vi "EI1050 Config.vi"(6 "Power Channel":i32=2, 7 "Enable Channels":i32[](array[numeric]), 8 "error in":errorcluster, 9 "Clock Channel":i32=1, 10 "Data Channel":i32, 11 "Handle In":i32) -> (0 "error out":errorcluster, 3 "Handle Out":i32)   [LabVIEW 2021]
panel:
  # "This array can be left empty if\nthere is only 1 EI-1050 and enable/disable\nis not needed."
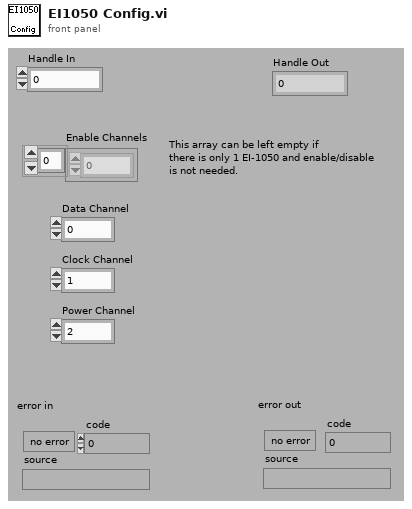
[diagram p1: front panel]
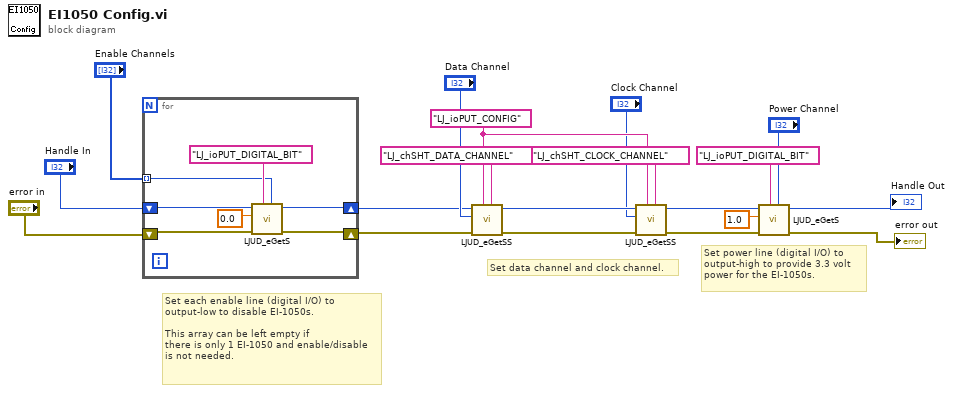
[diagram p0: block diagram]
diagram:
  w17 = "LJ_ioPUT_CONFIG"
  # "Set power line (digital I/O) to\noutput-high to provide 3.3 volt\npower for the EI-1050s."
  # "Set each enable line (digital I/O) to\noutput-low to disable EI-1050s.\n\nThis array can be left empty if\nthere is only 1 EI-1050 and enable/disable\nis not needed."
  # "Set data channel and clock channel."
  n1 = for {
    shift-right: [w23] -> w3
    shift-left: "error in" -> [w21]
    shift-right: [w24] -> w4
    shift-left: "Handle In" -> [w22]
    tunnel: "Enable Channels" -> [w20] mode=indexing
    n2 = call "LJUD_eGetS.vi"("Channel"=w20, "IOType"="LJ_ioPUT_DIGITAL_BIT", "error in"=w21, "Value Write"=0.0, "Handle In"=w22) -> ("error out"=w23:errorcluster, "Handle Out"=w24:i32)  [unwired: 4 in, 1 out]
  }
  n3 = call "LJUD_eGetSS.vi"("Channel"="LJ_chSHT_DATA_CHANNEL" ("IOType"), "IOType"=w17, "error in"=w3, "Value Write"="Data Channel", "Handle In"=w4) -> ("error out"=w13:errorcluster, "Handle Out"=w14:i32)  [unwired: 4 in, 1 out]
  n4 = call "LJUD_eGetSS.vi"("Channel"="LJ_chSHT_CLOCK_CHANNEL" ("IOType"), "IOType"=w17, "error in"=w13, "Value Write"="Clock Channel", "Handle In"=w14) -> ("error out"=w16:errorcluster, "Handle Out"=w15:i32)  [unwired: 4 in, 1 out]
  n5 = call "LJUD_eGetS.vi"("Channel"="Power Channel", "IOType"="LJ_ioPUT_DIGITAL_BIT", "error in"=w16, "Value Write"=1.0, "Handle In"=w15) -> ("error out"=→"error out":errorcluster, "Handle Out"=→"Handle Out":i32)  [unwired: 4 in, 1 out]
